vi "Arduino Move To Next Notch.vi"(5 "Ignore Alarm":bool, 7 "Distance":i32, 8 "error in":errorcluster, 9 "Homing Parameters":T1, 10 "Motor":i32, 11 "Addr":refnum<visa-resource-name>) -> (0 "error out":errorcluster, 2 "Actual distance":i32, 3 "Log":string)   [LabVIEW 2024, in "FW Arduino Control.lvclass"]
uses:
  FW Arduino Control.lvclass
  Filter Wheel Arduino Homing cluster.ctl
  da37c6a6-a1a6-4c15-8ebf-7ada4fc6adfa.vi
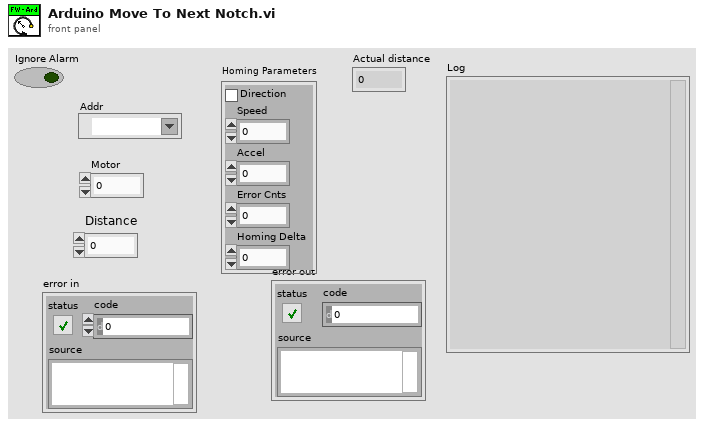
[diagram p1: front panel]
types:
  T1 = typedef "Filter Wheel Arduino Homing cluster.ctl" = cluster{"Direction":bool, "Speed":i32, "Accel":i32, "Error Cnts":i32, "Homing Delta":i32}
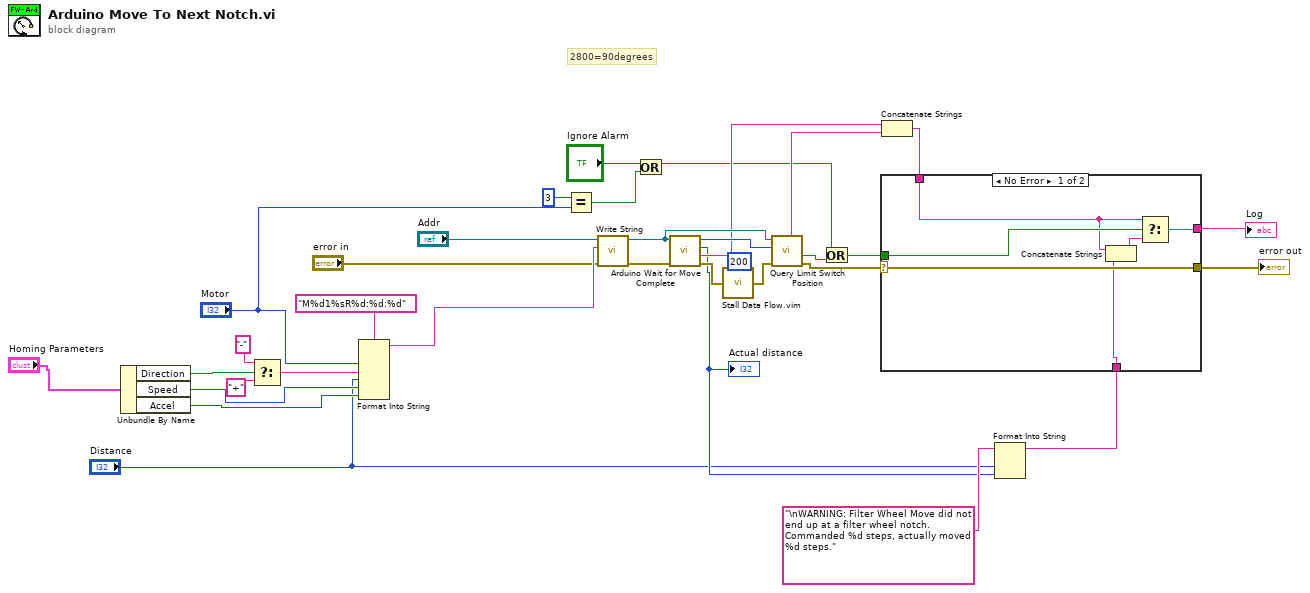
[diagram p0: block diagram]
diagram:
  # "2800=90degrees"
  n1 = Unbundle By Name("Homing Parameters") -> ("Direction"=w27:bool, "Speed"=w24:i32, "Accel"=w26:i32)
  n2 = Select(t="-", s=w27, f="+") -> (s? t:f=w30:string)
  n3 = Format Into String(format string="M%d1%sR%d:%d:%d", "Motor", w30, "Distance", w24, w26) -> (resulting string=w29:string)  [unwired: 2 in, 1 out]
  n4 = Equal?(x=3, y="Motor") -> (x = y?=w1:bool)
  n5 = call "Write String.vi"("error in (no error)"="error in", "String"=w29, "VISA resource name"="Addr") -> ("error out"=w25:errorcluster, "VISA resource name out"=w22:refnum<visa-resource-name>)  [unwired: 7 in]
  n6 = Or(x="Ignore Alarm", y=w1) -> (x .or. y?=w4:bool)
  n7 = call "Arduino Wait for Move Complete.vi"("error in (no error)"=w25, "reference"=w22) -> ("error out"=w23:errorcluster, "response"=w19:string, "distance"=w15:i32, "Motor"=w21:i32)  [unwired: 6 in]
  "Actual distance" <- w15
  n8 = call "Stall Data Flow.vim"("value in"=w23, "milliseconds to wait"=u32 200) -> ("value out"=w11:errorcluster)  [unwired: 1 out]
  n9 = call "Query Limit Switch Position.vi"("error in (no error)"=w11, "motor (0:n-1)"=w21, "VISA resource name"=w22) -> ("error out"=w17:errorcluster, "At Switch?"=w18:bool, "response"=w20:string)  [unwired: 4 in, 2 out]
  n10 = Or(x=w4, y=w18) -> (x .or. y?=w9:bool)
  n11 = Concatenate Strings(w19, w20) -> (w7:string)
  n12 = Format Into String(format string="\nWARNING: Filter Wheel Move did not end up at a filter wheel notch. Commanded %d steps, actually moved %d steps.", "Distance", w15) -> (resulting string=w13:string)  [unwired: 2 in, 1 out]
  n13 = case shown="No Error" w17 {
    selector: w17 -> [w40 w42]
    tunnel: w9 -> [w39 _]
    tunnel: w13 -> [w37 _]
    tunnel: [w40 w42] -> w12
    tunnel: w7 -> [w36 w41]
    tunnel: [w35 w41] -> w6
    frame No Error {
      n14 = Concatenate Strings(w36, w37) -> (w38:string)
      n15 = Select(t=w36, s=w39, f=w38) -> (s? t:f=w35:string)
    }
    frame Error {
    }
  }
  "error out" <- w12
  "Log" <- w6
